vi "ManipChangeState.vi"(2 "Reinit":bool, 3 "Instruction String":string) -> (0 "Error Out":errorcluster, 1 "Advance Trigger":bool)   [LabVIEW 2020]
doc: "This VI changes the robot's master state.\n\nParameters:\n1. state --> the robot's master state number"
uses:
  SafeParser_Integer.vi
  GlobalDriverStationCommands.vi
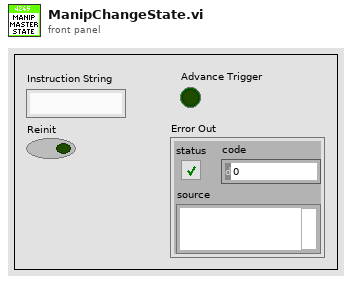
[diagram p1: front panel]
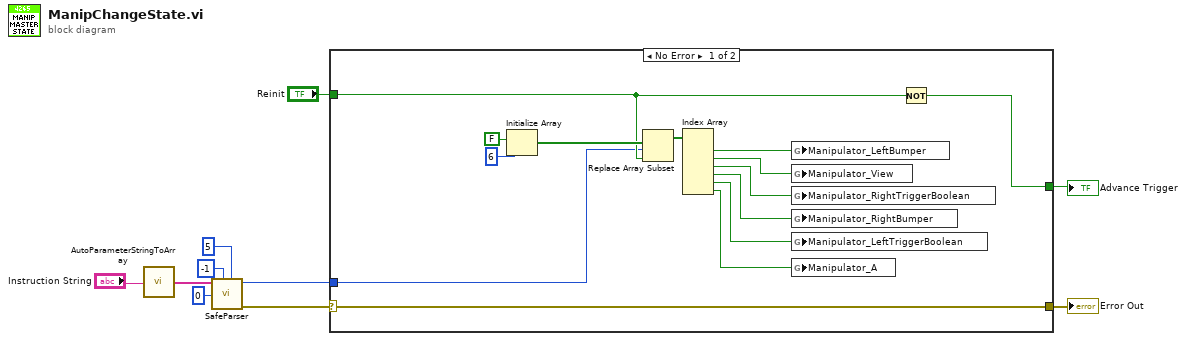
[diagram p0: block diagram]
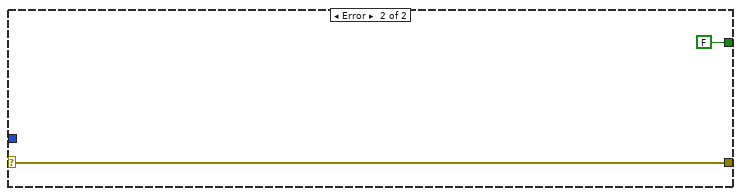
[diagram p2: hidden frame]
diagram:
  n1 = call "AutoParameterStringToArray.vi"("Parameter String"="Instruction String") -> ("Parsed Parameters"=w6:string[])
  n2 = call-poly "SafeParser.vi"("Maximum"=5, "Minimum"=-1, "Array Index"=0 ("Parameter Index"), "String Array"=w6) -> ("Error Out"=w8:errorcluster, "Typecast  Value"=w2:i32)  [unwired: 6 in]
  n3 = case shown="No Error" w8 {
    selector: w8 -> [w24 w26]
    tunnel: [w12 FALSE ("Advance Trigger")] -> w10
    tunnel: [w24 w26] -> w9
    tunnel: w2 -> [w11 _]
    tunnel: "Reinit" -> [w13 _]
    frame No Error {
      n4 = Initialize Array(FALSE, 6 ("dimension size")) -> (w22:bool[])
      n5 = Replace Array Subset(array=w22, new element=w13, index=w11) -> (w20:bool[])
      n6 = Index Array(array=w20) -> (element #1=w19:bool, element #2=w18:bool, element #3=w17:bool, element #4=w16:bool, element #5=w15:bool, element #6=w14:bool)  [unwired: 6 in]
      n7 = global write "GlobalDriverStationCommands.vi" "Manipulator_LeftBumper"(w19) -> ()
      n8 = global write "GlobalDriverStationCommands.vi" "Manipulator_View"(w18) -> ()
      n9 = global write "GlobalDriverStationCommands.vi" "Manipulator_RightTriggerBoolean"(w17) -> ()
      n10 = global write "GlobalDriverStationCommands.vi" "Manipulator_RightBumper"(w16) -> ()
      n11 = global write "GlobalDriverStationCommands.vi" "Manipulator_LeftTriggerBoolean"(w15) -> ()
      n12 = global write "GlobalDriverStationCommands.vi" "Manipulator_A"(w14) -> ()
      n13 = Not(x=w13) -> (.not. x?=w12:bool)
    }
    frame Error {
    }
  }
  "Advance Trigger" <- w10
  "Error Out" <- w9
